vi "GoToBallPlacementAllyTactic.vi"(7 "firstCall":bool, 8 "error in (no error)":errorcluster, 9 "Game in":refnum<class "Game.lvclass">, 10 "Robot":refnum<class "Robot.lvclass">, 11 "GoToBallPlacementAllyTactic in":refnum<class "GoToBallPlacementAllyTactic.lvclass">) -> (0 "error out":errorcluster, 2 "Robot out":refnum<class "Robot.lvclass">, 3 "GoToBallPlacementAllyTactic out":refnum<class "GoToBallPlacementAllyTactic.lvclass">)   [LabVIEW 2021, in "GoToBallPlacementAllyTactic.lvclass"]
uses:
  GoToBallPlacementAllyTactic.lvclass
  D:/RoboIme/horie/SSL_AI/Tactic_class/Tactic.lvclass
  Robot_class/Robot.lvclass
  Game_class/Game.lvclass
  StatesGoToBallPlacementAllyTactic.ctl
  Robot_class/tactics.ctl
  Tactic_class/Tactic.lvclass/Tactic.ctl
  Skillbook_class/Skillbook.lvclass/Skillbook.ctl
  Robot_class/robotKickToStates.ctl
  Robot_class/Robot.lvclass/Robot.ctl
  GoToBallPlacementAllyTactic.lvclass/GoToBallPlacementAllyTactic.ctl
  Skillbook_class/Read GoToNearBallPlacementSkill.vi
  Skillbook_class/Read PrepareToPositionBallPlacementSkill.vi
  Skillbook_class/Read KickToSkill.vi
  Tactic_class/Read Skillbook.vi
  Write States.vi
  Robot_class/Write tactic.vi
  Skillbook_class/Skillbook.lvclass
  GoToNearBallPlacementSkill_class/GoToNearBallPlacementSkill.lvclass
  PrepareToPositionBallPlacementSkill_class/PrepareToPositionBallPlacementSkill.lvclass
  KickToSkill_class/KickToSkill.lvclass
  Utilities_class/Utilities.lvclass
panel:
  out "x .or. y?":bool
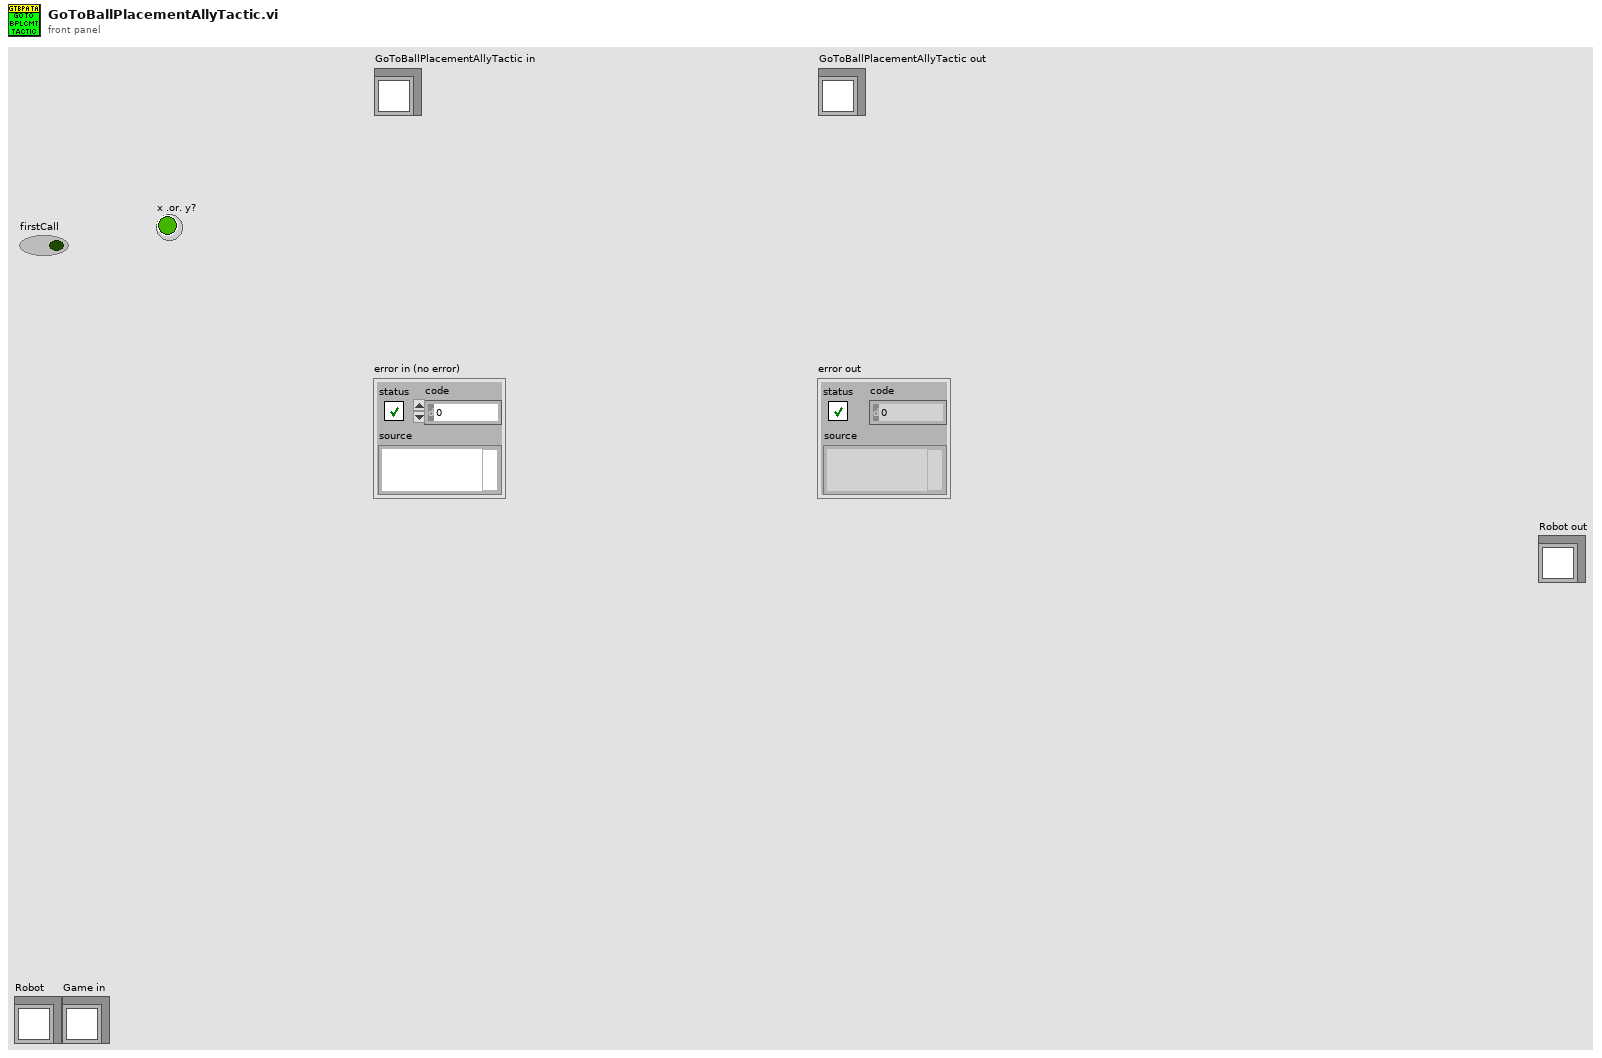
[diagram p1: front panel]
types:
  T1 = typedef "StatesGoToBallPlacementAllyTactic.ctl" = enum16{"GoToNearBall", "GoToBall", "PrepareToPositionBall", "Exit"}
  T2 = typedef "tactics.ctl" = enum16{"GoToBallPlacementPosition", "PlaceBall", "GoToBallPlacement", "5Robots", "BallPlacementEnemy", "ReceivePassInFuturePoint", "Roller", "PrepareRollToPassRollerGoTo", "PrepareRollToPassReceiverGoTo", "WaitRoll", "PositionToRoll", "PenaltyAttacker", "PassObserver", "PenaltyDefense", "TableReceiverTactic", "Test", "DefendGoal", "Marker", "FollowAttacker", "DefendArea", "Shoot", "AttackerAimGoal", "AttackerBallOutOfField", "AttackerBlock", "AttackerStop", "Duelist", "Halt", "ZigZag", "GoTo", "Timeout", "KickToBestRobot", "KickToPassReceiver", "PositionToReceivePass", "WaitPass"}
  T3 = typedef "robotKickToStates.ctl" = enum16{"shootFromDirect", "avoidCollideBall", "goToBackBall", "none", "walk", "turn", "oldKickToShoot", "oldKickToGoToBackBall", "shoot"}
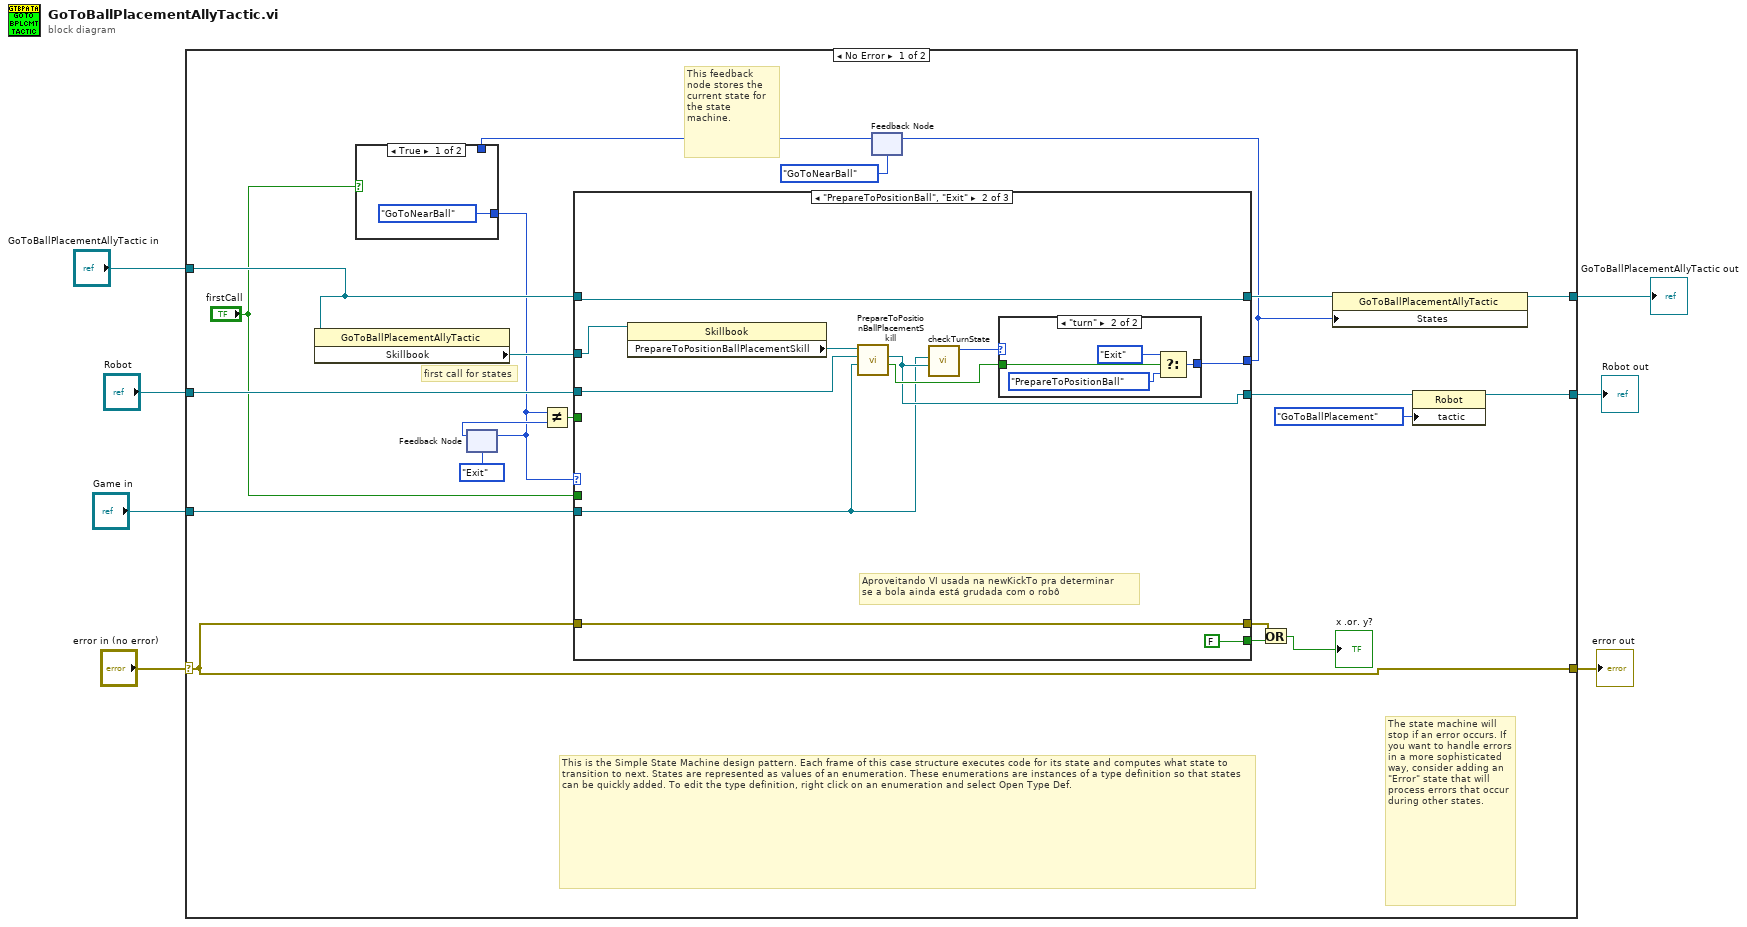
[diagram p0: block diagram]
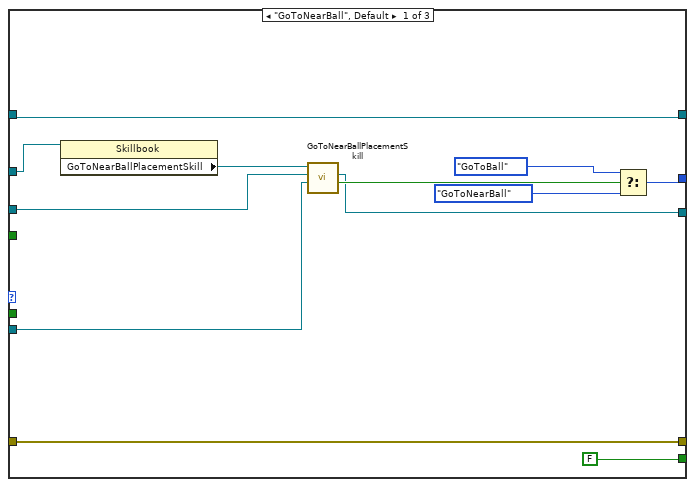
[diagram p3: hidden frame]
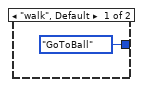
[diagram p4: hidden frame]
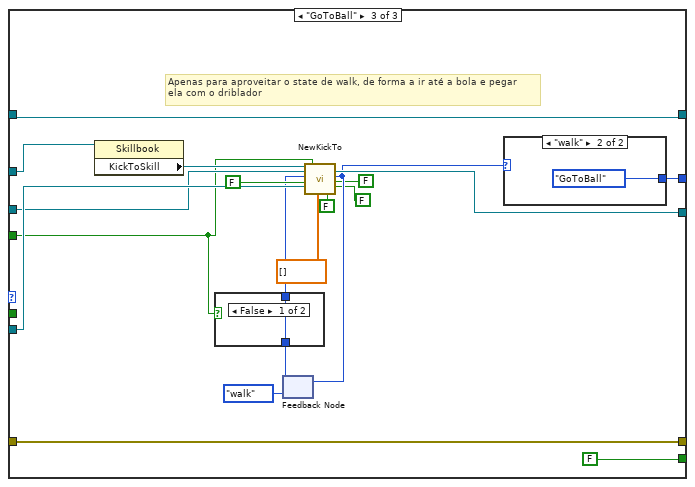
[diagram p5: hidden frame]
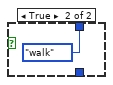
[diagram p6: hidden frame]
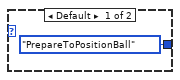
[diagram p7: hidden frame]
diagram:
  n1 = case shown="No Error" "error in (no error)" {
    selector: "error in (no error)" -> [w21 w83]
    tunnel: [w21 w83] -> w6
    tunnel: [w20 w82] -> w4
    tunnel: "GoToBallPlacementAllyTactic in" -> [w22 w82]
    tunnel: [w17 _] -> w3
    tunnel: "Robot" -> [w15 _]
    tunnel: "Game in" -> [w14 _]
    frame No Error {
      # "first call for states"
      # "The state machine will stop if an error occurs. If you want to handle errors in a more sophisticated way, consider adding an \"Error\" state that will process errors that occur during other states."
      # "This feedback node stores the current state for the state machine."
      # "This is the Simple State Machine design pattern. Each frame of this case structure executes code for its state and computes what state to transition to next. States are represented as values of an enumeration. These enumerations are instances of a type definition so that states can be quickly added. To edit the type definition, right click on an enumeration and select Open Type Def."
      n2 = property class="GoToBallPlacementAllyTactic"(reference=w22) -> ("Skillbook"=w25:refnum<class "Skillbook.lvclass">)  [unwired: 1 in, 2 out]
      n3 = feedback #1(StatesGoToBallPlacementAllyTactic."Exit" ("States")) -> (w10:T1)
      n4 = feedback #2(StatesGoToBallPlacementAllyTactic."GoToNearBall" ("States")) -> (w13:T1)
      n5 = case shown="True" "firstCall" {
        tunnel: [StatesGoToBallPlacementAllyTactic."GoToNearBall" ("States") w30] -> w9
        tunnel: w13 -> [_ w30]
        frame True {
        }
        frame False {
        }
      }
      n6 = feedback-in #1(w9) -> ()
      n7 = Not Equal?(x=w9, y=w10) -> (x != y?=w8:bool)
      n8 = case shown="\"PrepareToPositionBall\", \"Exit\"" w9 {
        tunnel: [FALSE ("Stop Loop?") FALSE ("Stop Loop?") FALSE ("Stop Loop?")] -> w27
        tunnel: w25 -> [w41 w52 w76]
        tunnel: w15 -> [w32 w44 w67]
        tunnel: [w33 w45 w72] -> w23
        tunnel: [w42 w53 w77] -> w24
        tunnel: w22 -> [w42 w53 w77]
        tunnel: w14 -> [w31 w43 w68]
        tunnel: [w40 w51 w75] -> w28
        tunnel: w21 -> [w40 w51 w75]
        tunnel: [w35 w47 w71] -> w18
        tunnel: "firstCall" -> [_ _ _]
        tunnel: w8 -> [_ _ w59]
        frame "GoToNearBall", Default {
          n9 = property class="Skillbook"(reference=w41) -> ("GoToNearBallPlacementSkill"=w38:refnum<class "GoToNearBallPlacementSkill.lvclass">)  [unwired: 1 in, 2 out]
          n10 = call "GoToNearBallPlacementSkill.vi"("Game"=w31, "Robot"=w32, "GoToNearBallPlacementSkill in"=w38) -> ("arrive"=w37:bool, "Robot out"=w33:refnum<class "Robot.lvclass">)  [unwired: 5 in, 2 out]
          n11 = Select(t=StatesGoToBallPlacementAllyTactic."GoToBall" ("States 2"), s=w37, f=StatesGoToBallPlacementAllyTactic."GoToNearBall" ("States 2")) -> (s? t:f=w35:T1)
        }
        frame "PrepareToPositionBall", "Exit" {
          # "Aproveitando VI usada na newKickTo pra determinar\nse a bola ainda está grudada com o robô"
          n12 = property class="Skillbook"(reference=w52) -> ("PrepareToPositionBallPlacementSkill"=w49:refnum<class "PrepareToPositionBallPlacementSkill.lvclass">)  [unwired: 1 in, 2 out]
          n13 = call "PrepareToPositionBallPlacementSkill.vi"("Game"=w43, "Robot"=w44, "PrepareToPositionBallPlacementSkill in"=w49) -> ("robotCanDoNextAction"=w48:bool, "Robot out"=w45:refnum<class "Robot.lvclass">)  [unwired: 5 in, 2 out]
          n14 = call "checkTurnState.vi"("Robot"=w45, "Game"=w43) -> ("robotKickState"=w46:T3)  [unwired: 9 in]
          n15 = case shown="\"turn\"" w46 {
            tunnel: w48 -> [_ w58]
            tunnel: [StatesGoToBallPlacementAllyTactic."GoToBall" ("States") w55] -> w47
            frame "walk", Default {
            }
            frame "turn" {
              n16 = Select(t=StatesGoToBallPlacementAllyTactic."Exit", s=w58, f=StatesGoToBallPlacementAllyTactic."PrepareToPositionBall" ("States")) -> (s? t:f=w55:T1)
            }
          }
        }
        frame "GoToBall" {
          # "Apenas para aproveitar o state de walk, de forma a ir até a bola e pegar\nela com o driblador"
          n17 = property class="Skillbook"(reference=w76) -> ("KickToSkill"=w73:refnum<class "KickToSkill.lvclass">)  [unwired: 1 in, 2 out]
          n18 = feedback #3(robotKickToStates."walk" ("State out")) -> (w60:T3)
          n19 = case shown="False" w59 {
            tunnel: [w78 robotKickToStates."walk" ("State out")] -> w61
            tunnel: w60 -> [w78 _]
            frame False {
            }
            frame True {
            }
          }
          n20 = call "NewKickTo.vi"("KickToSkill in"=w73, "Robot"=w67, "State in"=w61, "use criteria?"=FALSE, "Game"=w68, "firstCall?"=w59, "Target"=dbl[] [], "pass?"=FALSE, "chipKick ?"=FALSE, "ForceInGame"=FALSE) -> ("Robot out"=w72:refnum<class "Robot.lvclass">, "State out"=w70:T3)  [unwired: 6 in, 2 out]
          n21 = feedback-in #3(w70) -> ()
          n22 = case shown="\"walk\"" w70 {
            tunnel: [StatesGoToBallPlacementAllyTactic."PrepareToPositionBall" ("States") StatesGoToBallPlacementAllyTactic."GoToBall" ("States")] -> w71
            frame Default {
            }
            frame "walk" {
            }
          }
        }
      }
      n23 = feedback-in #2(w18) -> ()
      n24 = Or(x=w28, y=w27) -> (x .or. y?=→"x .or. y?":bool)
      n25 = property class="GoToBallPlacementAllyTactic"(reference=w24, "States"=w18) -> (reference out=w20:refnum<class "GoToBallPlacementAllyTactic.lvclass">)  [unwired: 1 in, 1 out]
      n26 = property class="Robot"(reference=w23, "tactic"=tactics."GoToBallPlacement") -> (reference out=w17:refnum<class "Robot.lvclass">)  [unwired: 1 in, 1 out]
    }
    frame Error {
    }
  }
  "error out" <- w6
  "GoToBallPlacementAllyTactic out" <- w4
  "Robot out" <- w3
